vi "Powersumpply.vi"() -> ()   [LabVIEW 2022 SP3]
panel:
  out "read buffer":string
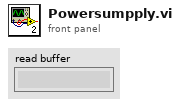
[diagram p1: front panel]
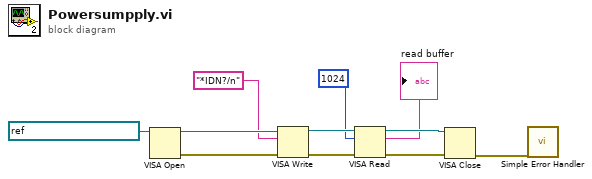
[diagram p0: block diagram]
diagram:
  n1 = VISA Open(VISA resource name=refnum<visa-resource-name> "GPIB0::10::INSTR") -> (VISA resource name=w10:refnum<visa-resource-name>, error out=w5:errorcluster)  [unwired: 4 in]
  n2 = VISA Write(VISA resource name=w10, write buffer="*IDN?/n", error in (no error)=w5) -> (VISA resource name out=w9:refnum<visa-resource-name>, error out=w6:errorcluster)  [unwired: 1 out]
  n3 = VISA Read(VISA resource name=w9, byte count=u32 1024, error in (no error)=w6) -> (VISA resource name out=w8:refnum<visa-resource-name>, read buffer=→"read buffer":string, error out=w7:errorcluster)  [unwired: 1 out]
  n4 = VISA Close(VISA resource name=w8, error in (no error)=w7) -> (error out=w1:errorcluster)
  n5 = call <vilib>:"Simple Error Handler.vi"("error in (no error)"=w1) -> ()  [unwired: 4 in, 5 out]
